vi "数据显示 (子VI).vi"(11 "Array输入":refnum<vi>) -> (3 "Table":string[][](table) caption="数据显示")   [LabVIEW 2016]
uses:
  <vilib>/Utility/miscctls.llb/LVPointTypeDef.ctl
panel:
  in  "切换主界面":bool
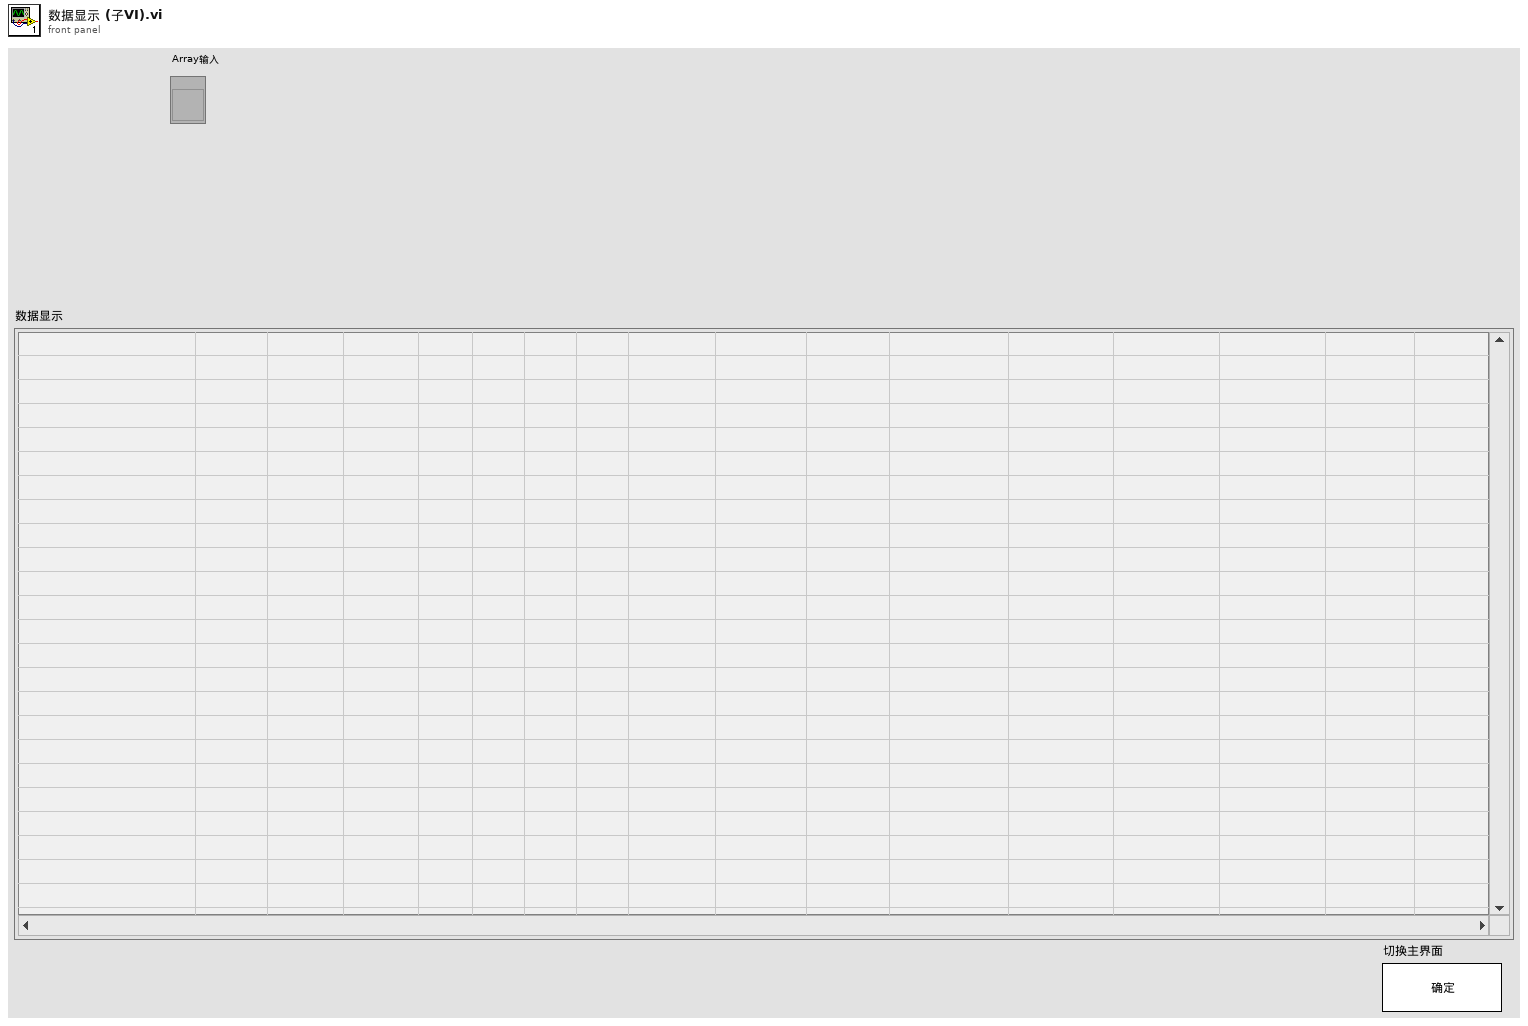
[diagram p1: front panel]
types:
  T1 = typedef "LVPointTypeDef.ctl" = cluster{"Horizontal":i16, "Vertical":i16}
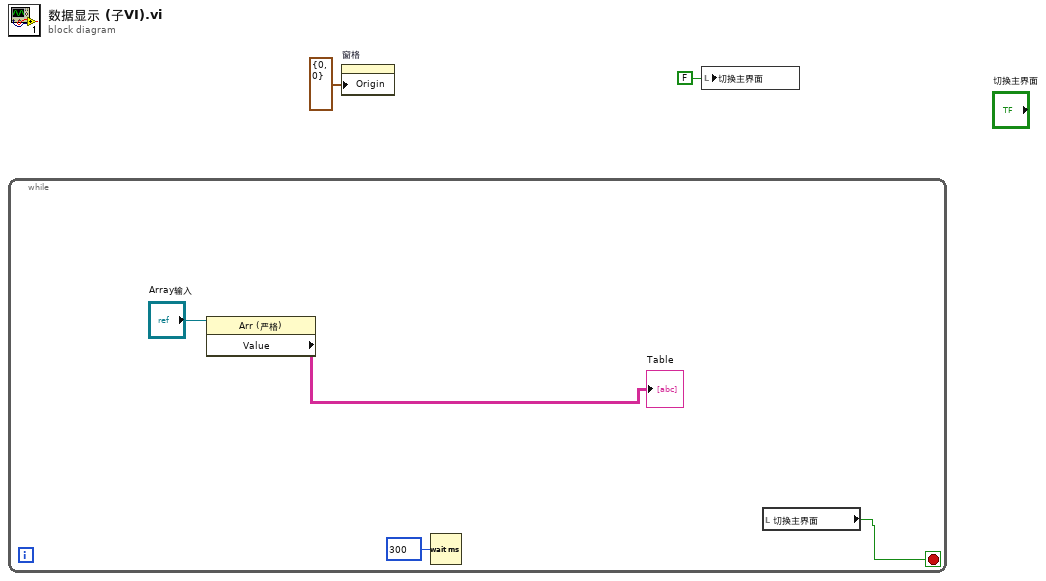
[diagram p0: block diagram]
diagram:
  n1 = while {
    stop <- w3 stop-if-true
    n2 = property class="Arr (严格)"(reference="Array输入") -> ("Value"=→"Table":string[][])  [unwired: 1 in, 2 out]
    n3 = Wait (ms)(milliseconds to wait=u32 300 ("等待时间（毫秒）")) -> ()  [unwired: 1 out]
    n4 = local read "切换主界面"() -> (w3:bool)
  }
  n5 = property on="窗格" class="Pane"("Origin"=T1 {"Horizontal"=0, "Vertical"=0} ("原点")) -> ()  [unwired: 2 in, 2 out]
  n6 = local write "切换主界面"(FALSE ("切换主界面")) -> ()
